vi "4 - QDSM Machine as method.vi"   [LabVIEW 2015]
uses:
  Child Actor/Child Actor.lvclass
  Parent Message/Parent Message.lvclass
  State/Parent Actor.lvclass/Parent Actor.ctl
  State/Parent Actor.lvclass
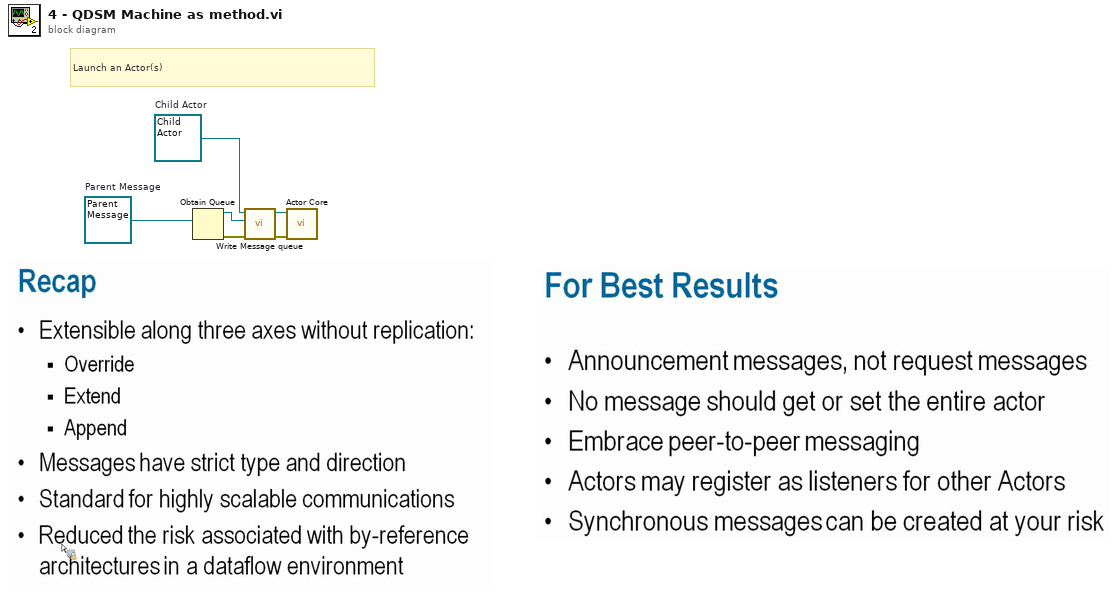
[diagram p0: block diagram]
diagram:
  w4 = refnum<class "Parent Message.lvclass"> refnum  # Parent Message
  w5 = refnum<class "Child Actor.lvclass"> refnum  # Child Actor
  # "Launch an Actor(s)"
  n1 = Obtain Queue(element data type=w4) -> (queue out=w3:refnum<queue>, error out=w2:errorcluster)  [unwired: 4 in, 1 out]
  n2 = call "Write Message queue.vi"("error in (no error)"=w2, "Message queue"=w3, "Parent Actor in"=w5) -> ("error out"=w1:errorcluster, "Parent Actor out"=w6:refnum<class "Child Actor.lvclass">)  [unwired: 7 in]
  n3 = call-dynamic "Actor Core.vi"("error in (no error)"=w1, "Child Actor in"=w6) -> ()  [unwired: 8 in, 2 out]
